vi "SV Continuous Swept-Sine THD.vi"(0 "scaled signals [EU]":waveform(dbl)[](array[waveform]), 1 "desired units":T4, 2 "reset? (F)":bool, 7 "maximum harmonic":i32=-1, 9 "harmonics to visualize":i32[](array[numeric]), 11 "error in (no error)":errorcluster, 12 "buffer settings":T2 {"buffer mode" items=["Infinite length", "Last block data", "Custom"]}, 13 "zero delay? (F)":bool) -> (3 "unit labels":T1(array[cluster]), 4 "scaled signals out [EU]":waveform(dbl)[](array[waveform]), 6 "THD":cluster{"frequency":dbl[], "amplitude":dbl[]}[](array[cluster]) {"amplitude" format="%.2f"; "frequency" format="%.2f"}, 8 "harmonic components":T3(array[cluster]), 15 "error out":errorcluster)   [LabVIEW 2017, in "SoundVib_ContSweptSine.lvlib"]
doc: "Computes the total harmonic distortion (THD) and harmonic values of the input signals by performing a continuous swept-sine measurement."
uses:
  <vilib>/addons/Sound and Vibration/svt_Continuous Swept Sine/SoundVib_ContSweptSine.lvlib
  <vilib>/addons/_NISVFA/_Shared subVIs/Controls/sv_Buffer XY Settings.ctl
  <vilib>/Analysis/1siggen.llb/Ramp Pattern by Samples.vi
  <vilib>/Analysis/NI_AALBase.lvlib
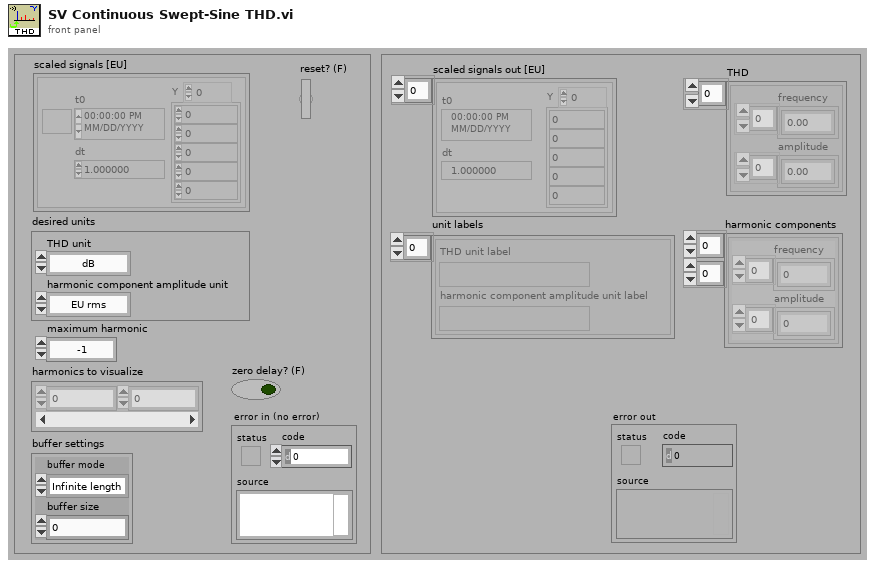
[diagram p1: front panel]
types:
  T1 = cluster{"THD unit label":string, "harmonic component amplitude unit label":string}[]
  T2 = typedef "sv_Buffer XY Settings.ctl" = cluster{"buffer mode":u16, "buffer size":dbl}
  T3 = cluster{"frequency":dbl[], "amplitude":dbl[]}[][]
  T4 = cluster{"THD unit":enum16{"dB", "linear ratio", "%"}, "harmonic component amplitude unit":enum16{"EU rms", "EU peak", "EU peak-peak", "dB ref fund"}}
  T5 = typedef "svc_Resampled Channel Info.ctl" = cluster{"channel name":string, "description":string, " channel info":T6}
  T6 = typedef "svc_Channel Info.ctl" = cluster{"sensor sensitivity":dbl, "engineering units":T7, "dB reference":dbl, "custom label":string, "weighting filter":T8, "pregain":dbl}
  T7 = typedef "svc_Engineering Units Text Ring.ctl" = u16
  T8 = typedef "svc_Weighting Filter Text Ring.ctl" = u16
  T9 = typedef "OAT Position Info.ctl" = cluster{"positions [s]":dbl[], "samples/rev":dbl}
  T10 = cluster{"time/rev/freq":dbl[], "magnitude":dbl[]}[][]
  T11 = typedef "svc_Spectrum Info.ctl" = cluster{"channel name":string, "description":string, "x-axis units":T12, "spectral info":cluster{"spectrum type":T13, "linear/dB":enum16{"linear", "dB"}, "window":u16, "window size":i32, "FFT size":i32}, "engineering units":T7, "custom label":string, "dB reference [EU]":dbl, "peak units":enum16{"rms", "peak", "peak-peak"}, "weighting filter":T8, "spectral density?":bool, "unit label":string, "spectrum skewed?":bool, "complimentary spectrum units":T14}
  T12 = typedef "svc_X-Axis Units.ctl" = u16
  T13 = typedef "svc_Spectrum Type.ctl" = enum16{"FFT Spectrum [complex]", "Amplitude [Magnitude]", "Power [Magnitude^2]", "Cross Spectrum [complex]", "Frequency Response [Complex]"}
  T14 = typedef "svc_Complimentary Spectrum Units.ctl" = enum16{"none", "radians", "degrees", "cycles", "imaginary"}
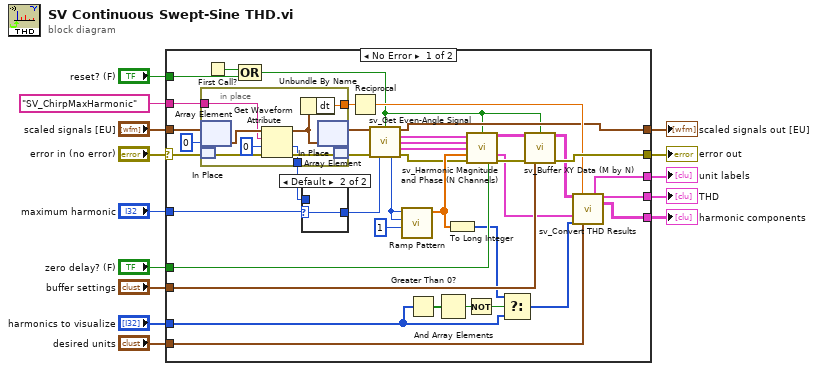
[diagram p0: block diagram]
diagram:
  n1 = case shown="No Error" "error in (no error)" {
    selector: "error in (no error)" -> [w29 w65]
    tunnel: [w40 w65] -> w13
    tunnel: [w35 _] -> w12
    tunnel: "harmonics to visualize" -> [w20 _]
    tunnel: [w33 _] -> w8
    tunnel: "scaled signals [EU]" -> [w31 w64]
    tunnel: [w23 w64] -> w9
    tunnel: "desired units" -> [w36 _]
    tunnel: [w34 _] -> w3
    tunnel: "buffer settings" -> [w42 _]
    tunnel: "zero delay? (F)" -> [w49 _]
    tunnel: "reset? (F)" -> [w47 _]
    tunnel: "maximum harmonic" -> [w18 _]
    tunnel: "SV_ChirpMaxHarmonic" ("name") -> [w16 _]
    frame No Error {
      n2 = in-place {
        in-place-border: [w63] -> w27
        in-place-border: w16 -> [w57]
        in-place-border: [w56] -> w15
        n3 = in-place-array #1(w31, 0) -> (w61:waveform(dbl))
        n4 = in-place-match #2(w29) -> (w59:errorcluster)
        n5 = Get Waveform Attribute(4:w59, 5:0, 6:w57, 7:w61) -> (0:w58:errorcluster, 1:w56:i32, 3:w60:waveform(dbl))  [unwired: 1 out]
        n6 = Unbundle By Name(w60) -> ("dt"=w63:dbl)
        n7 = in-place-array #1(w60) -> (w30:waveform(dbl)[])  [unwired: 1 out]
        n8 = in-place-match #2(w58) -> (w28:errorcluster)
      }
      n9 = First Call?() -> (First Call?: T/F=w48:bool)
      n10 = Compound Arithmetic op=OR(w48, w47) -> (w22:bool)
      n11 = case shown="Default" w18 {
        selector: w18 -> [_ w55]
        tunnel: [w54 w55] -> w17
        tunnel: w15 -> [w54 _]
        frame ..1 {
        }
        frame Default {
        }
      }
      n12 = Reciprocal(x=w27) -> (1/x=w26:dbl)
      n13 = call <vilib>:"sv_Get Even-Angle Signal.vi"("data to process"=w30, "reset?"=w22, "error in (no error)"=w28, "maximum harmonic"=w17) -> ("data to process out"=w23:waveform(dbl)[], "even-angle signals"=w53:cluster{"r0":dbl, "dr":dbl, "Y":dbl[]}[], "even-angle channel info"=w52:T5[], "even-angle position info"=w51:T9, "actual maximum harmonic"=w24:i32, "error out"=w32:errorcluster)  [unwired: 6 in]
      n14 = call-poly <vilib>:"Ramp Pattern.vi"("start"=1, "end"=w24, "samples"=w24) -> ("Ramp Pattern"=w44:dbl[])  [unwired: 7 in, 1 out]
      n15 = Greater Than 0?(x=w20) -> (x > 0?=w46:bool[])
      n16 = And Array Elements(Boolean array=w46) -> (logical AND=w45:bool)
      n17 = To Long Integer(number=w44) -> (32bit integer=w21:i32[])
      n18 = Not(x=w45) -> (.not. x?=w19:bool)
      n19 = call <vilib>:"sv_Harmonic Magnitude and Phase (N Channels).vi"("even-angle signals"=w53, "reset? (F)"=w22, "even-angle channel info"=w52, "even-angle position info"=w51, "orders to compute (1.0)"=w44, "error in (no error)"=w32, "zero delay? (F)"=w49) -> ("magnitudes [RMS]"=w43:T10, "magnitudes info"=w38:T11[], "error out"=w41:errorcluster)  [unwired: 5 in, 1 out]
      n20 = Select(t=w21, s=w19, f=w20) -> (s? t:f=w37:i32[])
      n21 = call <vilib>:"sv_Buffer XY Data (M by N).vi"("XY signals"=w43, "reset? (F)"=w22, "error in (no error)"=w41, "buffer settings"=w42) -> ("buffered XY signals"=w39:cluster{"X":dbl[], "Y":dbl[]}[][], "error out"=w40:errorcluster)  [unwired: 10 in]
      n22 = call <vilib>:"sv_Convert THD Results.vi"("Magnitudes"=w39, "acquisition sample rate [Hz]"=w26, "magnitudes info"=w38, "harmonics to visualize"=w37, "desired units"=w36) -> ("unit labels"=w34:T1, "THD"=w35:cluster{"frequency":dbl[], "amplitude":dbl[]}[], "harmonic components"=w33:T3)  [unwired: 8 in]
    }
    frame Error {
    }
  }
  "error out" <- w13
  "THD" <- w12
  "scaled signals out [EU]" <- w9
  "harmonic components" <- w8
  "unit labels" <- w3
